vi "DeleteSubVI.vi"(8 "error in (no error)":errorcluster, 11 "SubVI in":refnum<vi>) -> (0 "error out":errorcluster)   [LabVIEW 2011]
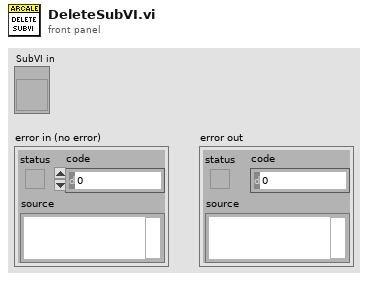
[diagram p1: front panel]
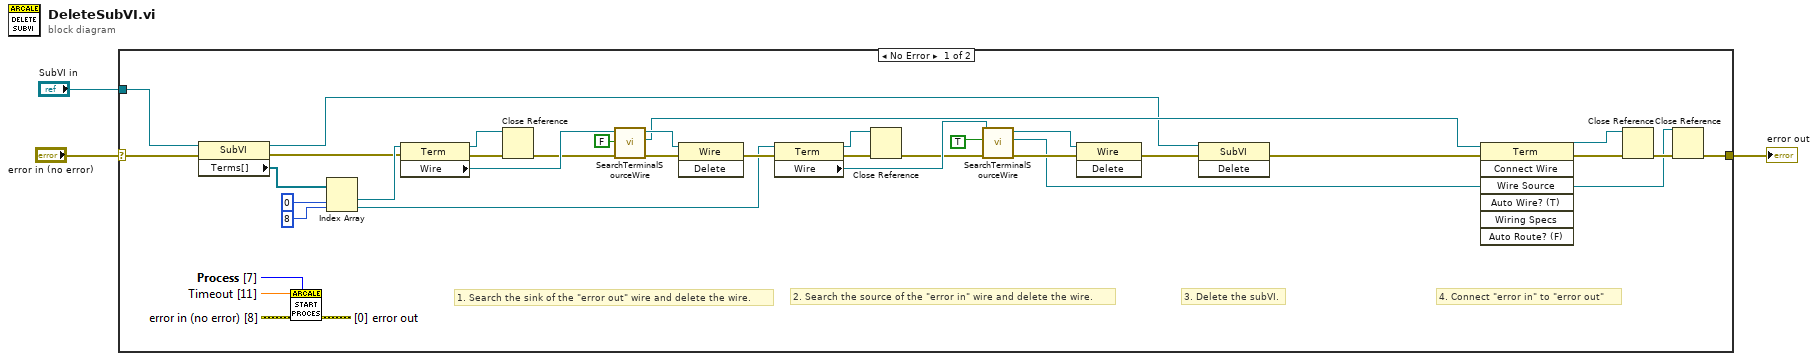
[diagram p0: block diagram]
diagram:
  n1 = case shown="No Error" "error in (no error)" {
    selector: "error in (no error)" -> [w19 w36]
    tunnel: [w6 w36] -> w3
    tunnel: "SubVI in" -> [w18 _]
    frame No Error {
      # "4. Connect \"error in\" to \"error out\""
      # "3. Delete the subVI."
      # "2. Search the source of the \"error in\" wire and delete the wire."
      # "1. Search the sink of the \"error out\" wire and delete the wire."
      n2 = property class="SubVI"(reference=w18, error in=w19) -> (reference out=w22:refnum<vi>, error out=w17:errorcluster, "Terms[]"=w35:refnum<vi>[])
      n3 = Index Array(array=w35, index #1=0 ("index"), index #2=8 ("index")) -> (element #1=w23:refnum<vi>, element #2=w25:refnum<vi>)
      n4 = property class="Term"(reference=w23, error in=w17) -> (reference out=w12:refnum<vi>, error out=w14:errorcluster, "Wire"=w28:refnum<vi>)
      n5 = Close Reference(reference=w12, error in (no error)=w14) -> (error out=w13:errorcluster)
      n6 = call "SearchTerminalSourceWire.vi"("error in (no error)"=w13, "Source?"=FALSE, "Refnum Wire In"=w28) -> ("error out"=w31:errorcluster, "Terminal Refnum"=w27:refnum<vi>, "Refnum Wire Out"=w30:refnum<vi>)  [unwired: 6 in]
      n7 = invoke class="Wire" method="Delete"(reference=w30, error in=w31) -> (error out=w32:errorcluster)  [unwired: 1 in, 2 out]
      n8 = property class="Term"(reference=w25, error in=w32) -> (reference out=w11:refnum<vi>, error out=w10:errorcluster, "Wire"=w29:refnum<vi>)
      n9 = Close Reference(reference=w11, error in (no error)=w10) -> (error out=w9:errorcluster)
      n10 = call "SearchTerminalSourceWire.vi"("error in (no error)"=w9, "Source?"=TRUE, "Refnum Wire In"=w29) -> ("error out"=w33:errorcluster, "Terminal Refnum"=w4:refnum<vi>, "Refnum Wire Out"=w34:refnum<vi>)  [unwired: 6 in]
      n11 = invoke class="Wire" method="Delete"(reference=w34, error in=w33) -> (error out=w16:errorcluster)  [unwired: 1 in, 2 out]
      n12 = invoke class="SubVI" method="Delete"(reference=w22, error in=w16) -> (error out=w15:errorcluster)  [unwired: 1 in, 2 out]
      n13 = invoke class="Term" method="Connect Wire"(reference=w27, error in=w15, "Wire Source"=w4) -> (reference out=w5:refnum<vi>, error out=w8:errorcluster)  [unwired: 4 in, 5 out]
      n14 = Close Reference(reference=w5, error in (no error)=w8) -> (error out=w7:errorcluster)
      n15 = Close Reference(reference=w4, error in (no error)=w7) -> (error out=w6:errorcluster)
    }
    frame Error {
    }
  }
  "error out" <- w3
